vi "zad_10.vi"() -> ()   [LabVIEW 2024]
uses:
  State_10.ctl
  Data_10.ctl
panel:
  out "error out":errorcluster
  in  "error in":errorcluster
  in  "Draught level [ml]":dbl(slide) scale=0.0..50.0
  in  "Drink beer":bool
  in  "No more drinking":bool
  out "Glass":cluster{dbl, dbl}(slide) scale=0.0..500.0
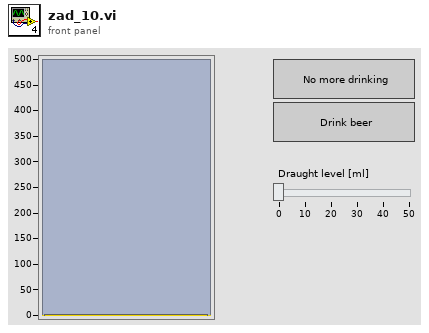
[diagram p1: front panel]
types:
  T1 = typedef "State_10.ctl" = enum16{"Init", "Idle", "Beer level update", "Drink beer", "Reset", "Drunk enought?", "Stop", "Error"}
  T2 = typedef "Data_10.ctl" = cluster{"Beer level":dbl, "Intendet level":dbl, "Number of beers":dbl, "Reset?":bool}
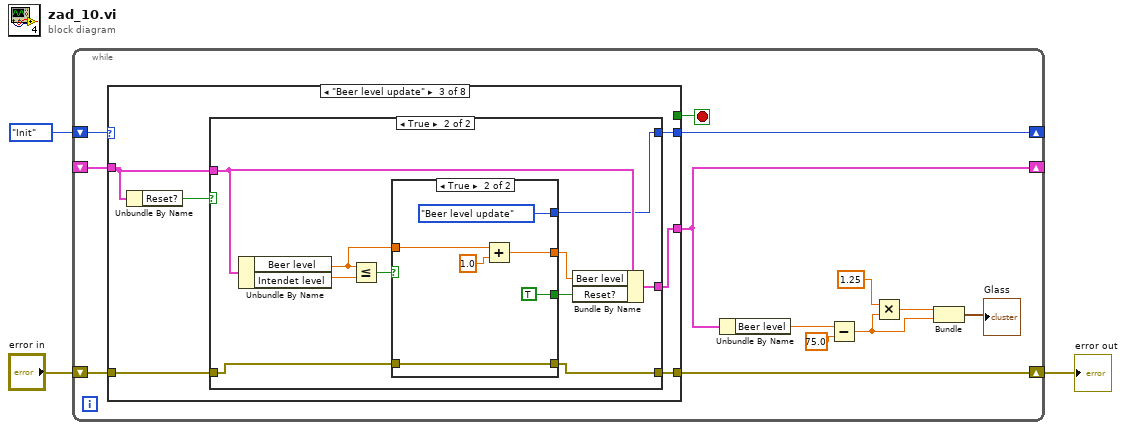
[diagram p0: block diagram]
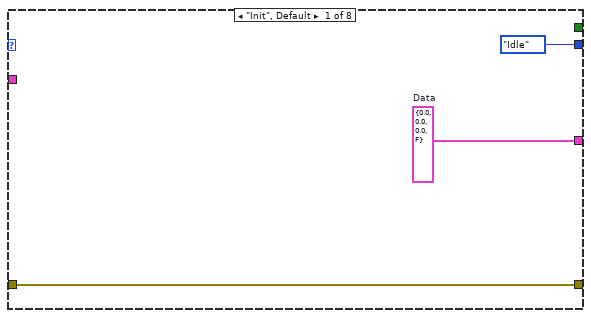
[diagram p2: hidden frame]
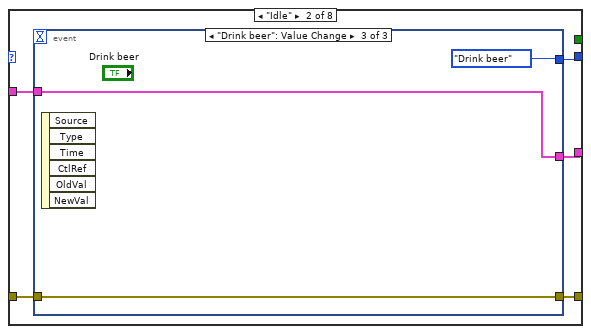
[diagram p3: hidden frame]
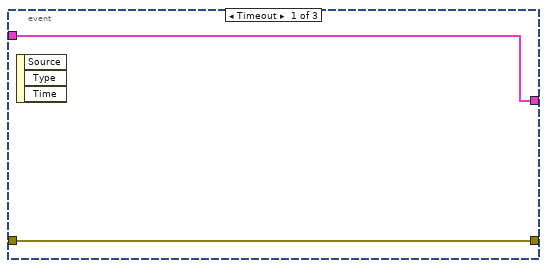
[diagram p4: hidden frame]
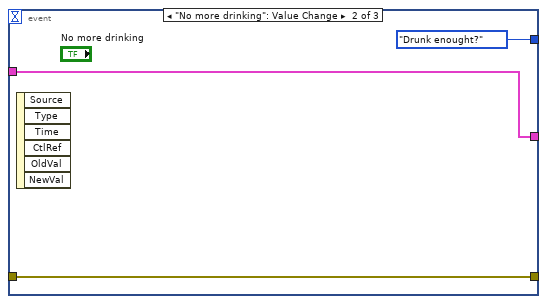
[diagram p5: hidden frame]
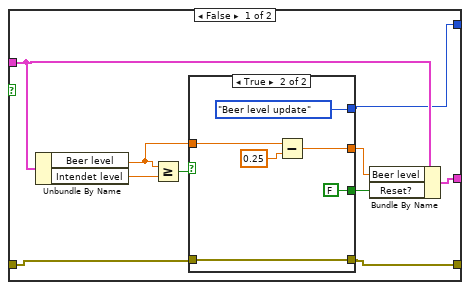
[diagram p6: hidden frame]
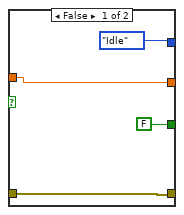
[diagram p7: hidden frame]
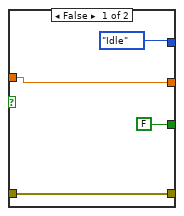
[diagram p8: hidden frame]
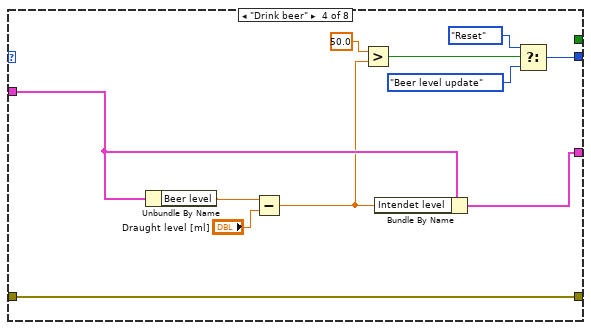
[diagram p9: hidden frame]
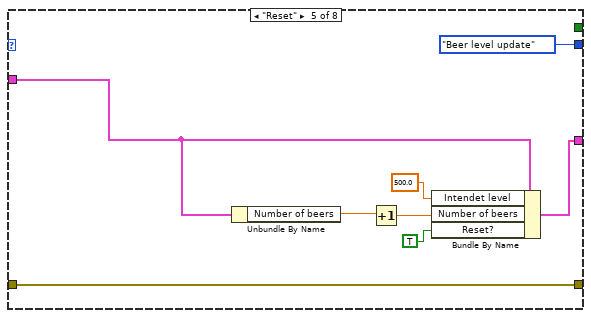
[diagram p10: hidden frame]
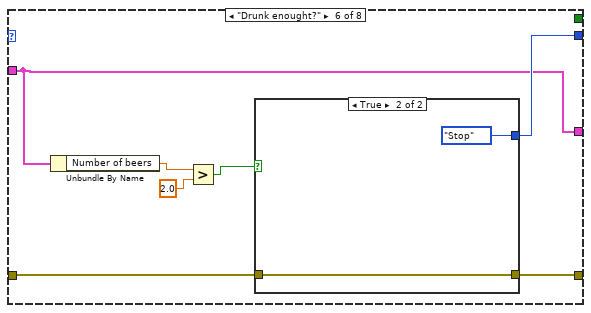
[diagram p11: hidden frame]
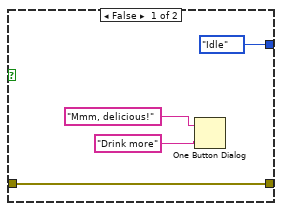
[diagram p12: hidden frame]
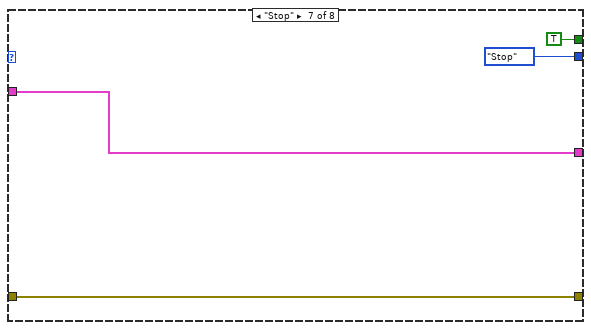
[diagram p13: hidden frame]
diagram:
  n1 = while {
    shift-right: [w14] -> _
    shift-left: State_10."Init" -> [w16]
    shift-right: [w10] -> _
    shift-left: _ -> [w13]
    shift-right: [w11] -> w1
    shift-left: "error in" -> [w12]
    stop <- w15 stop-if-true
    n2 = case shown="\"Beer level update\"" w16 {
      selector: w16 -> [_ _ _ _ _ _ _ w116]
      tunnel: [_ _ _ _ _ _ TRUE _] -> w15
      tunnel: [State_10."Idle" w20 w34 w86 State_10."Beer level update" w104 State_10."Stop" w116] -> w14
      tunnel: [w17 w22 w33 w79 w91 w101 w112 w117] -> w10
      tunnel: w13 -> [_ w21 w38 w81 w94 w101 w112 w117]
      tunnel: [w19 w24 w36 w89 w97 w103 w111 w115] -> w11
      tunnel: w12 -> [w19 w23 w35 w89 w97 w102 w111 w115]
      frame "Init", Default {
        w17 = T2 {"Beer level"=0.0, "Intendet level"=0.0, "Number of beers"=0.0, "Reset?"=FALSE}  # Data
      }
      frame "Idle" {
        n3 = event shown="[2] \"Drink beer\": Value Change" {
          selector: _ -> [_ _ _]
          dyn-events: _ -> [_ _ _]
          timeout: _ -> [_ _ _]
          tunnel: [w26 w28 w30] -> w24
          tunnel: w23 -> [w26 w28 w30]
          tunnel: [w25 w27 w32] -> w22
          tunnel: w21 -> [w25 w27 w32]
          tunnel: [_ State_10."Drunk enought?" State_10."Drink beer"] -> w20
          event Timeout {
            n4 = event-data() -> ()  [unwired: 1 in, 3 out]
          }
          event "No more drinking": Value Change {
            n5 = event-data() -> ()  [unwired: 1 in, 6 out]
          }
          event "Drink beer": Value Change {
            n6 = event-data() -> ()  [unwired: 1 in, 6 out]
          }
        }
      }
      frame "Beer level update" {
        n7 = Unbundle By Name(w38) -> ("Reset?"=w37:bool)
        n8 = case shown="True" w37 {
          tunnel: w38 -> [w46 w66]
          tunnel: [w41 w60] -> w36
          tunnel: w35 -> [w40 w59]
          tunnel: [w45 w62] -> w34
          tunnel: [w39 w61] -> w33
          frame False {
            n9 = Unbundle By Name(w46) -> ("Beer level"=w43:dbl, "Intendet level"=w44:dbl)
            n10 = Greater Or Equal?(x=w43, y=w44) -> (x >= y?=w42:bool)
            n11 = case shown="True" w42 {
              tunnel: w43 -> [w51 w55]
              tunnel: [w51 w54] -> w48
              tunnel: [FALSE ("Reset?") FALSE ("Reset?")] -> w47
              tunnel: [State_10."Idle" State_10."Beer level update"] -> w45
              tunnel: [w49 w53] -> w41
              tunnel: w40 -> [w49 w53]
              frame False {
              }
              frame True {
                n12 = Subtract(x=w55, y=0.25) -> (x-y=w54:dbl)
              }
            }
            n13 = Bundle By Name(cluster=w46, "Beer level"=w48, "Reset?"=w47) -> (w39:T2)
          }
          frame True {
            n14 = Unbundle By Name(w66) -> ("Beer level"=w65:dbl, "Intendet level"=w67:dbl)
            n15 = Less Or Equal?(x=w65, y=w67) -> (x <= y?=w68:bool)
            n16 = case shown="True" w68 {
              tunnel: w65 -> [w71 w78]
              tunnel: [w71 w76] -> w64
              tunnel: [FALSE ("Reset?") TRUE ("Reset?")] -> w63
              tunnel: [State_10."Idle" State_10."Beer level update"] -> w62
              tunnel: [w69 w73] -> w60
              tunnel: w59 -> [w69 w73]
              frame False {
              }
              frame True {
                n17 = Add(x=w78, y=1.0) -> (x+y=w76:dbl)
              }
            }
            n18 = Bundle By Name(cluster=w66, "Beer level"=w64, "Reset?"=w63) -> (w61:T2)
          }
        }
      }
      frame "Drink beer" {
        n19 = Unbundle By Name(w81) -> ("Beer level"=w83:dbl)
        n20 = Subtract(x=w83, y="Draught level [ml]") -> (x-y=w80:dbl)
        n21 = Greater?(x=50.0, y=w80) -> (0:w85:bool)
        n22 = Bundle By Name(cluster=w81, "Intendet level"=w80) -> (w79:T2)
        n23 = Select(t=State_10."Reset", s=w85, f=State_10."Beer level update") -> (s? t:f=w86:T1)
      }
      frame "Reset" {
        n24 = Unbundle By Name(w94) -> ("Number of beers"=w90:dbl)
        n25 = Increment(x=w90) -> (x+1=w95:dbl)
        n26 = Bundle By Name(cluster=w94, "Intendet level"=500.0, "Number of beers"=w95, "Reset?"=TRUE) -> (w91:T2)
      }
      frame "Drunk enought?" {
        n27 = Unbundle By Name(w101) -> ("Number of beers"=w99:dbl)
        n28 = Greater?(x=w99, y=2.0) -> (0:w98:bool)
        n29 = case shown="True" w98 {
          tunnel: [State_10."Idle" State_10."Stop"] -> w104
          tunnel: [w108 w109] -> w103
          tunnel: w102 -> [w108 w109]
          frame False {
            n30 = One Button Dialog(message="Mmm, delicious!", button name ("OK")="Drink more") -> ()  [unwired: 1 out]
          }
          frame True {
          }
        }
      }
      frame "Stop" {
      }
      frame "Error" {
      }
    }
    n31 = Unbundle By Name(w10) -> ("Beer level"=w5:dbl)
    n32 = Subtract(x=w5, y=75.0) -> (x-y=w6:dbl)
    n33 = Multiply(x=1.25, y=w6) -> (x*y=w9:dbl)
    n34 = Bundle(w9, w6) -> (→"Glass":cluster{dbl, dbl})  [unwired: 1 in]
  }
  "error out" <- w1
